vi "Manipulator Controller.vi"   [LabVIEW 2018]
uses:
  <vilib>/Rock Robotics/WPI/Joystick/WPI_JoystickDeviceEnum.ctl
  Manipulator Controller Global.vi
types:
  T1 = typedef "WPI_JoystickDeviceEnum.ctl" = enum16{"USB 0", "USB 1", "USB 2", "USB 3", "USB 4", "USB 5"}
  T2 = typedef "WPI_JoystickDevRef.ctl" = cluster{"Device":T1}
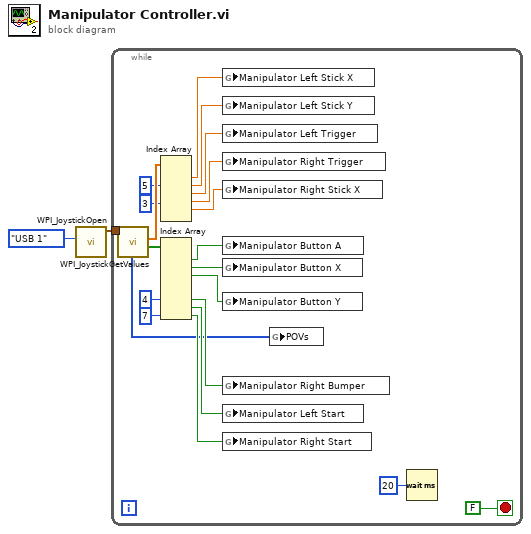
[diagram p0: block diagram]
diagram:
  n1 = call <vilib>:"WPI_JoystickOpen.vi"("JoystickDevice"=WPI_JoystickDeviceEnum."USB 1") -> ("JoystickDevRef"=w1:T2)  [unwired: 10 in]
  n2 = while {
    tunnel: w1 -> [w23]
    stop <- FALSE stop-if-true
    n3 = call <vilib>:"WPI_JoystickGetValues.vi"("JoystickDevRef"=w23) -> ("Buttons"=w21:bool[], "Axes"=w22:dbl[], "POVs"=w3:i16[])  [unwired: 6 in, 2 out]
    n4 = Index Array(array=w22, index #2=5 ("index"), index #4=3 ("index")) -> (element #1=w20:dbl, element #2=w19:dbl, element #3=w18:dbl, element #4=w17:dbl, element #5=w16:dbl)  [unwired: 4 in, 1 out]
    n5 = Index Array(array=w21, index #6=4 ("index"), index #8=7 ("index")) -> (element #1=w15:bool, element #2=w14:bool, element #3=w13:bool, element #6=w12:bool, element #7=w11:bool, element #8=w10:bool)  [unwired: 6 in, 2 out]
    n6 = global write "Manipulator Controller Global.vi" "Manipulator Left Stick X"(w20) -> ()
    n7 = global write "Manipulator Controller Global.vi" "Manipulator Left Stick Y"(w19) -> ()
    n8 = global write "Manipulator Controller Global.vi" "Manipulator Left Trigger"(w18) -> ()
    n9 = global write "Manipulator Controller Global.vi" "Manipulator Right Trigger"(w17) -> ()
    n10 = global write "Manipulator Controller Global.vi" "Manipulator Right Stick X"(w16) -> ()
    n11 = global write "Manipulator Controller Global.vi" "Manipulator Button A"(w15) -> ()
    n12 = global write "Manipulator Controller Global.vi" "Manipulator Button X"(w14) -> ()
    n13 = global write "Manipulator Controller Global.vi" "Manipulator Button Y"(w13) -> ()
    n14 = global write "Manipulator Controller Global.vi" "Manipulator Right Bumper"(w12) -> ()
    n15 = global write "Manipulator Controller Global.vi" "Manipulator Left Start"(w11) -> ()
    n16 = global write "Manipulator Controller Global.vi" "Manipulator Right Start"(w10) -> ()
    n17 = global write "Manipulator Controller Global.vi" "POVs"(w3) -> ()
    n18 = Wait (ms)(milliseconds to wait=u32 20) -> ()  [unwired: 1 out]
  }
